vi "Execute Publication Policy.vi"(7 "Default PublicationPolicy":refnum<class "IPublicationPolicy.lvclass">, 9 "Last Publish Time":timestamp, 10 "Last Published Value":variant, 11 "PublishRequest":refnum<class "PublishRequest.lvclass">) -> (0 "error out (Reject Publication)":errorcluster, 1 "Publication Time":timestamp, 2 "Value to Publish":variant)   [LabVIEW 2020, in "IMediator.lvlib" / "PublishRequest.lvclass"]
doc: "此方法决定是否发送或以其他方式处理新数据值。该策略由订阅者设置和维护。Topic Actor不知道任何策略细节，它只是将新值传入。如果此方法内部出现故障，Topic Acton必须假设侦听器不再有效（死亡/不可恢复），并应将其从订阅服务器列表中删除。"
uses:
  PublishRequest.lvclass
  IPublicationPolicy/IPublicationPolicy.lvclass
  PublishRequest.lvclass/PublishRequest.ctl
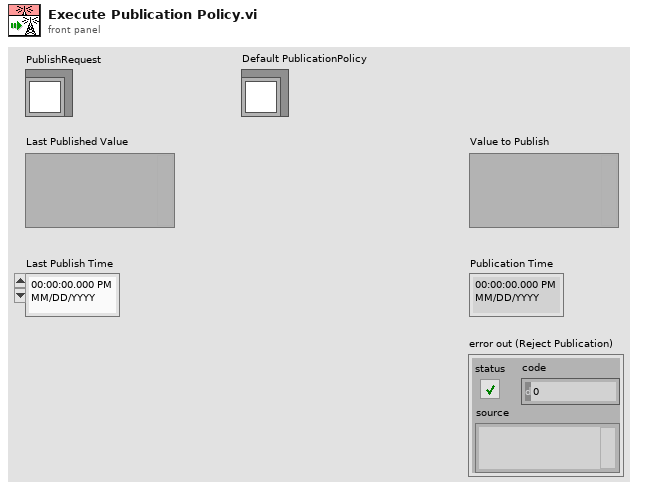
[diagram p1: front panel]
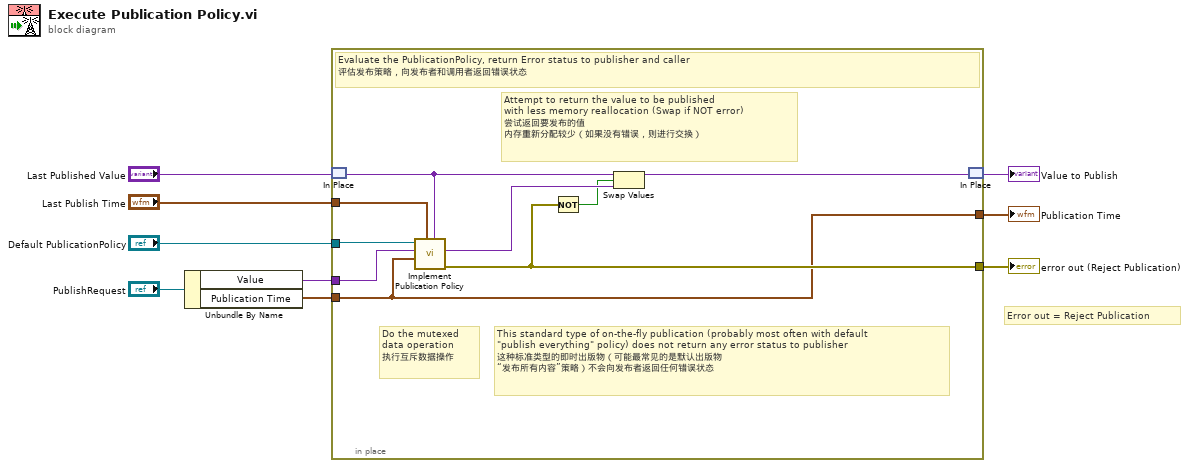
[diagram p0: block diagram]
diagram:
  # "Error out = Reject Publication"
  n1 = Unbundle By Name("PublishRequest") -> ("Value"=w3:variant, "Publication Time"=w2:timestamp)
  n2 = in-place {
    in-place-border: [w11] -> w8
    in-place-border: "Default PublicationPolicy" -> [w15]
    in-place-border: w3 -> [w14]
    in-place-border: w2 -> [w10]
    in-place-border: "Last Publish Time" -> [w12]
    in-place-border: [w10] -> w1
    # "This standard type of on-the-fly publication (probably most often with default\n\"publish everything\" policy) does not return any error status to publisher\n这种标准类型的即时出版物（可能最常见的是默认出版物\n“发布所有内容”策略）不会向发布者返回任何错误状态"
    # "Do the mutexed\ndata operation\n执行互斥数据操作"
    # "Attempt to return the value to be published\nwith less memory reallocation (Swap if NOT error)\n尝试返回要发布的值\n内存重新分配较少（如果没有错误，则进行交换）"
    # "Evaluate the PublicationPolicy, return Error status to publisher and caller\n评估发布策略，向发布者和调用者返回错误状态"
    n3 = in-place-match #1("Last Published Value") -> (w13:variant)
    n4 = call-dynamic "Implement Publication Policy.vi"("Last Published Value"=w13, "Last Published Time"=w12, "New Value Time"=w10, "New Value"=w14, "PublicationPolicy"=w15) -> ("error out (Reject Publication)"=w11:errorcluster, "Value to Publish"=w17:variant)  [unwired: 5 in]
    n5 = Not(x=w11) -> (.not. x?=w16:bool)
    n6 = Swap Values(12:w13, 13:w16, 14:w17) -> (1:w18:variant)  [unwired: 1 out]
    n7 = in-place-match #1(w18) -> (→"Value to Publish":variant)
  }
  "error out (Reject Publication)" <- w8
  "Publication Time" <- w1
